vi "dot product.vi"(1 "y":dbl[][](array[numeric]), 2 "x":dbl[][](array[numeric])) -> (0 "dot(x,y)":dbl[][](array[numeric]))   [LabVIEW 2020]
uses:
  <vilib>/Analysis/baseanly.llb/Real A x B.vi
  <vilib>/Analysis/Matrix/Numeric/Conversions/Array To Matrix - RA2.vi
  <vilib>/Analysis/Matrix/Numeric/Conversions/Matrix To Array - RM.vi
  <vilib>/Analysis/Matrix/NI_Matrix.lvlib
  <vilib>/Analysis/NI_AALBase.lvlib
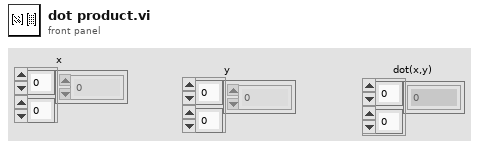
[diagram p1: front panel]
types:
  T1 = typedef "NI_Matrix.lvlib/RealMatrix.ctl" = dbl[][]
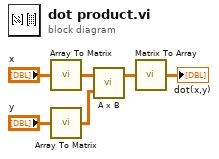
[diagram p0: block diagram]
diagram:
  n1 = call-poly <vilib>:"Array To Matrix.vi"("Real 2D Array"="x") -> ("Real Matrix"=w1:T1)
  n2 = call-poly <vilib>:"Array To Matrix.vi"("Real 2D Array"="y") -> ("Real Matrix"=w2:T1)
  n3 = call-poly <vilib>:"A x B.vi"("B"=w2, "A"=w1) -> ("A x B"=w3:T1)  [unwired: 1 out]
  n4 = call-poly <vilib>:"Matrix To Array.vi"("Real Matrix"=w3) -> ("Real 2D Array"=→"dot(x,y)":dbl[][])
